vi "lua_insert.vi"(8 "error in (no error)":errorcluster, 10 "index":i32, 11 "lua_state_p":u64) -> (0 "error out":errorcluster, 3 "lua_state_p out":u64)   [LabVIEW 2020, in "lua.dll.lvlib"]
uses:
  lua.dll.lvlib
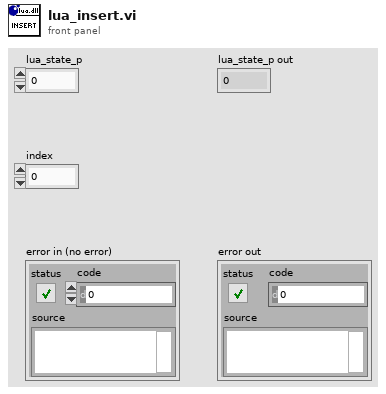
[diagram p1: front panel]
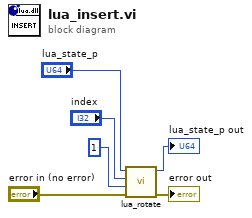
[diagram p0: block diagram]
diagram:
  n1 = call "lua_rotate.vi"("error in (no error)"="error in (no error)", "n"=1, "index"="index", "lua_state_p"="lua_state_p") -> ("error out"=→"error out":errorcluster, "lua_state_p out"=→"lua_state_p out":u64)  [unwired: 6 in]
